vi "Bias SubVI.vi"(10 "Array":dbl[][](array[numeric]), 11 "B0":dbl[](array[numeric])=[1.0, 1.0, 1.0]) -> (1 "Bias GyrZ":T1={"Bias Error Chart"=[14892.335499998195], "Bias"=[0.0, 0.0, 0.0], "Final Bias Error"=0.0, "data processed"=[]}, 2 "Bias GyrY":T1={"Bias Error Chart"=[14892.335499998195], "Bias"=[0.0, 0.0, 0.0], "Final Bias Error"=0.0, "data processed"=[]}, 3 "Bias GyrX":T1={"Bias Error Chart"=[14892.335499998195], "Bias"=[0.0, 0.0, 0.0], "Final Bias Error"=0.0, "data processed"=[]})   [LabVIEW 2021, in "IMU Processing.lvlib"]
uses:
  IMU Processing.lvlib
  Bias.ctl
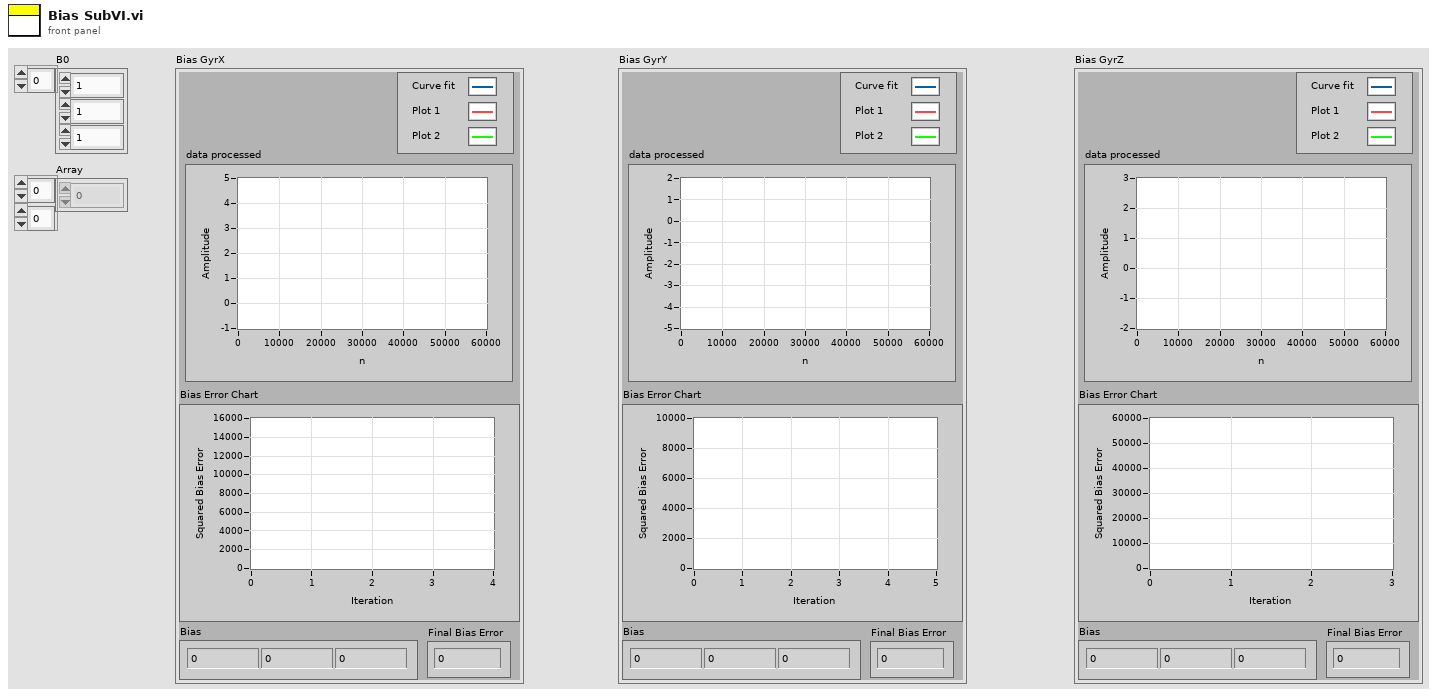
[diagram p1: front panel]
types:
  T1 = typedef "Bias.ctl" = cluster{"Bias Error Chart":dbl[], "Bias":dbl[], "Final Bias Error":dbl, "data processed":cluster{dbl[]}[]}
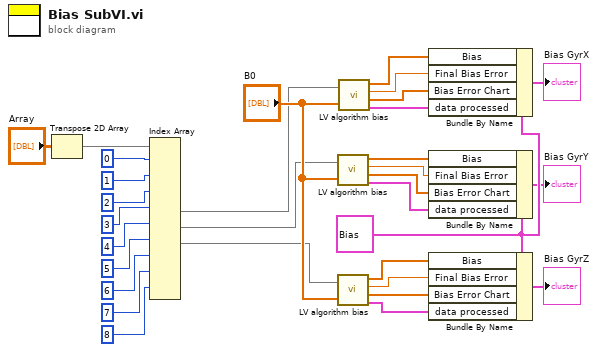
[diagram p0: block diagram]
diagram:
  w27 = T1 {"Bias Error Chart"=[14892.335499998195], "Bias"=[], "Final Bias Error"=14892.335499998195, "data processed"=[{[]}]} ("Bias")
  n1 = Transpose 2D Array(2D array="Array") -> (transposed array=w2:dbl[][])
  n2 = Index Array(array=w2, index (row) #1=0 ("index (row)"), index (row) #2=1 ("index (row)"), index (row) #3=2 ("index (row)"), index (row) #4=3 ("index (row)"), index (row) #5=4 ("index (row)"), index (row) #6=5 ("index (row)"), index (row) #7=6 ("index (row)"), index (row) #8=7 ("index (row)"), index (row) #9=8 ("index (row)")) -> (element #4=w26:dbl[], element #5=w20:dbl[], element #6=w25:dbl[])  [unwired: 9 in, 6 out]
  n3 = call "LV algorithm bias.vi"("data"=w20, "B0"="B0") -> ("B new"=w16:dbl[], "Error B"=w17:dbl, "Interation Error Graph"=w18:dbl[], "data processed"=w29:cluster{dbl[]}[])
  n4 = call "LV algorithm bias.vi"("data"=w25, "B0"="B0") -> ("B new"=w21:dbl[], "Error B"=w22:dbl, "Interation Error Graph"=w23:dbl[], "data processed"=w30:cluster{dbl[]}[])
  n5 = call "LV algorithm bias.vi"("data"=w26, "B0"="B0") -> ("B new"=w15:dbl[], "Error B"=w14:dbl, "Interation Error Graph"=w13:dbl[], "data processed"=w28:cluster{dbl[]}[])
  n6 = Bundle By Name(cluster=w27, "Bias"=w15, "Final Bias Error"=w14, "Bias Error Chart"=w13, "data processed"=w28) -> (→"Bias GyrX":T1)
  n7 = Bundle By Name(cluster=w27, "Bias"=w16, "Final Bias Error"=w17, "Bias Error Chart"=w18, "data processed"=w29) -> (→"Bias GyrY":T1)
  n8 = Bundle By Name(cluster=w27, "Bias"=w21, "Final Bias Error"=w22, "Bias Error Chart"=w23, "data processed"=w30) -> (→"Bias GyrZ":T1)
